vi "Create Dispatcher.vi"(7 "framework options":T1, 8 "error in (no error)":errorcluster, 10 "Plugins":refnum<class "Plugin.lvclass">[](array[class]), 11 "Framework in":refnum<class "Framework.lvclass">) -> (0 "error out":errorcluster, 2 "Dispatcher Thread":refnum<class "Dispatcher Thread.lvclass">, 3 "Framework out":refnum<class "Framework.lvclass">)   [LabVIEW 2017, in "DSF Core.lvlib" / "Framework.lvclass"]
uses:
  Framework.lvclass
  Plugin/Plugin.lvclass
  Thread/Dispatcher/Dispatcher Thread.lvclass
  Framework Options.ctl
  Typedefs/DSF FIFO Options.ctl
  Thread/DSF Thread Options.ctl
  Typedefs/DSF Plugin Options.ctl
  Typedefs/DSF Performance Options.ctl
  Thread/Thread Settings.ctl
  Framework.lvclass/Framework.ctl
  Thread/Thread.lvclass
  DSF Core.lvlib
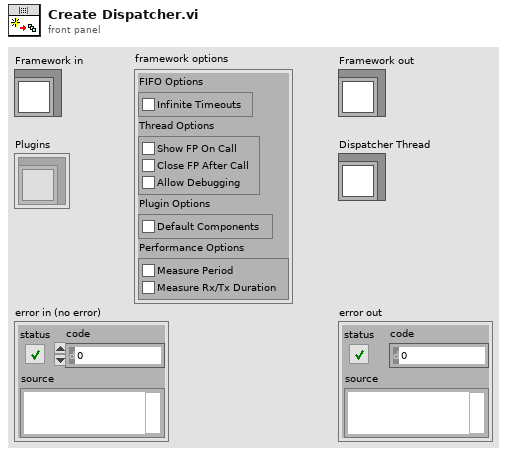
[diagram p1: front panel]
types:
  T1 = typedef "DSF Core.lvlib/Framework.lvclass/Framework Options.ctl" = cluster{"FIFO Options":T2, "Thread Options":T3, "Plugin Options":T4, "Performance Options":T5}
  T2 = typedef "DSF Core.lvlib/DSF FIFO Options.ctl" = cluster{"Infinite Timeouts":bool}
  T3 = typedef "DSF Core.lvlib/DSF Thread Options.ctl" = cluster{"Show FP On Call":bool, "Close FP After Call":bool, "Allow Debugging":bool}
  T4 = typedef "DSF Core.lvlib/DSF Plugin Options.ctl" = cluster{"Default Components":bool}
  T5 = typedef "DSF Core.lvlib/DSF Performance Options.ctl" = cluster{"Measure Period":bool, "Measure Rx/Tx Duration":bool}
  T6 = typedef "DSF Core.lvlib/Thread.lvclass/Thread Settings.ctl" = cluster{"Priority":u16, "Processor":i32, "ID":i32}
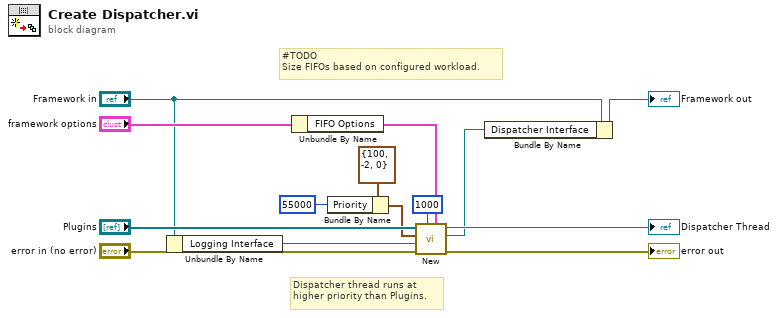
[diagram p0: block diagram]
diagram:
  # "Dispatcher thread runs at higher priority than Plugins."
  # "#TODO\nSize FIFOs based on configured workload."
  n1 = Unbundle By Name("Framework in") -> ("Logging Interface"=w1:refnum<class "Logging Interface.lvclass">)
  n2 = Unbundle By Name("framework options") -> ("FIFO Options"=w3:T2)
  n3 = Bundle By Name(cluster=T6 {"Priority"=100, "Processor"=-2, "ID"=0} ("Thread Parameters"), "Priority"=u16 55000 ("priority (100)")) -> (w4:T6)
  n4 = call "New.vi"("FIFO Options"=w3, "fifo depths"=u32 1000, "error in (no error)"="error in (no error)", "Logging Interface"=w1, "Thread Parameters"=w4, "Plugins"="Plugins") -> ("error out"=→"error out":errorcluster, "Dispatcher Interface"=w10:refnum<class "Dispatcher Interface.lvclass">, "Dispatcher Thread"=→"Dispatcher Thread":refnum<class "Dispatcher Thread.lvclass">)  [unwired: 3 in]
  n5 = Bundle By Name(cluster="Framework in", "Dispatcher Interface"=w10) -> (→"Framework out":refnum<class "Framework.lvclass">)
